vi "getGridElements.vi"(8 "error in (no error)":errorcluster, 11 "TransactionList in":refnum<class "TransactionList.lvclass">) -> (0 "error out":errorcluster, 2 "Grid Rows":string[][](array[string]), 3 "TransactionList out":refnum<class "TransactionList.lvclass">)   [LabVIEW 2020, in "TransactionList.lvclass"]
uses:
  TransactionList.lvclass
  TransactionList.lvclass/TransactionList.ctl
  Transaction/Transaction.lvclass
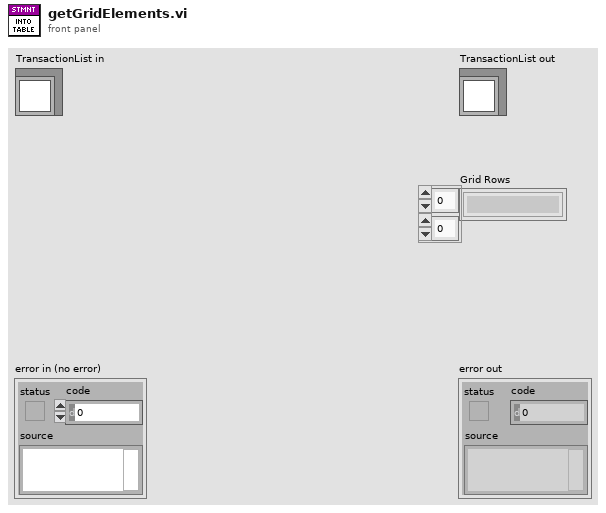
[diagram p1: front panel]
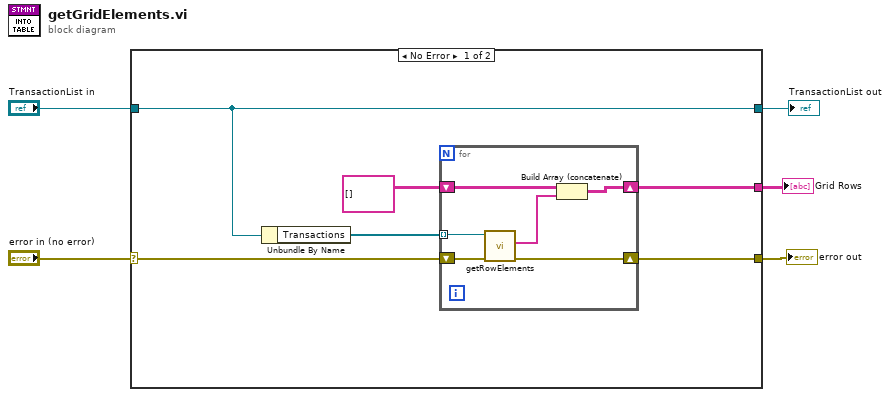
[diagram p0: block diagram]
diagram:
  n1 = case shown="No Error" "error in (no error)" {
    selector: "error in (no error)" -> [w8 w19]
    tunnel: [w11 w19] -> w4
    tunnel: [w10 w18] -> w2
    tunnel: "TransactionList in" -> [w10 w18]
    tunnel: [w6 _] -> w1
    frame No Error {
      n2 = Unbundle By Name(w10) -> ("Transactions"=w9:refnum<class "Transaction.lvclass">[])
      n3 = for {
        tunnel: w9 -> [w15] mode=indexing
        shift-right: [w12] -> w11
        shift-left: w8 -> [w14]
        shift-right: [w16] -> w6
        shift-left: string[][] [] ("Table Row") -> [w17]
        n4 = call-dynamic "getRowElements.vi"("error in (no error)"=w14, "Transaction in"=w15) -> ("error out"=w12:errorcluster, "Table Row"=w13:string[])  [unwired: 7 in, 1 out]
        n5 = Build Array (concatenate)(w17, w13) -> (w16:string[][])
      }
    }
    frame Error {
    }
  }
  "error out" <- w4
  "TransactionList out" <- w2
  "Grid Rows" <- w1
